vi "GEOM_Bin1DetReadMode.vi"(9 "detectors":T1[](array[typedef]), 10 "Amplifiers":T2[](array[typedef]) {"fliped" items=["none", "horizontal", "vertical"]; "type" items=["LL", "LR", "UL", "UR"]}) -> (1 "detectors out":T1[](array[typedef]))   [LabVIEW 2016]
uses:
  GEOM_Amplifier.ctl
  GEOM_AmpType.ctl
  GEOM_ROI.ctl
  GEOM_Coords.ctl
  GEOM_DetSummaryStruct.ctl
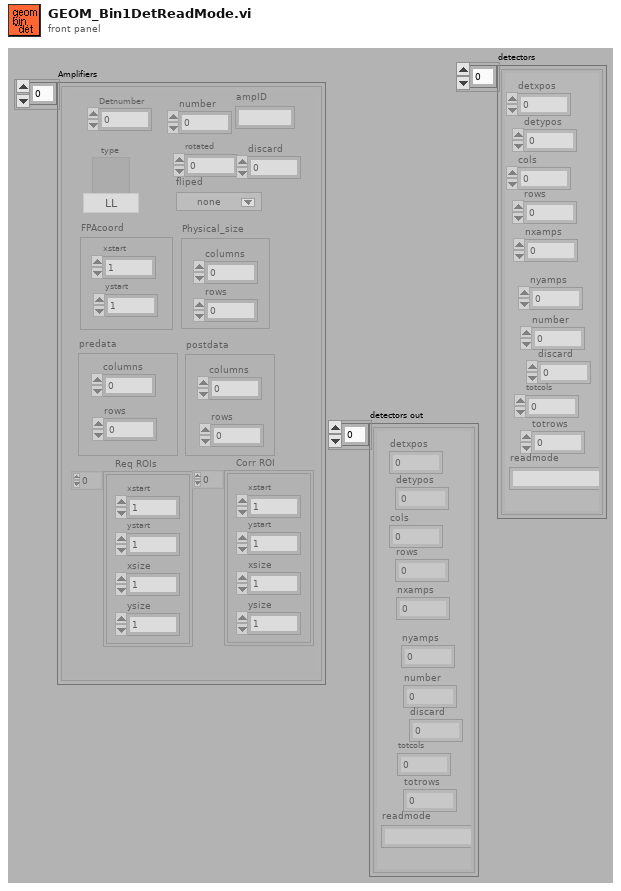
[diagram p1: front panel]
types:
  T1 = typedef "GEOM_DetSummaryStruct.ctl" = cluster{"detxpos":i32, "detypos":i32, "cols":i32, "rows":i32, "nxamps":i32, "nyamps":i32, "number":i32, "discard":i32, "totcols":i32, "totrows":i32, "readmode":string}
  T2 = typedef "GEOM_Amplifier.ctl" = cluster{"number":i32, "type":T3, "rotated":i16, "fliped":u16, "FPAcoord":cluster{"xstart":i32, "ystart":i32}, "Physical_size":cluster{"columns":i32, "rows":i32}, "predata":cluster{"columns":i32, "rows":i32}, "postdata":cluster{"columns":i32, "rows":i32}, "Req ROIs":T4, "Corr ROI":T4, "Detnumber":i32, "ampID":string, "discard":i32}
  T3 = typedef "GEOM_AmpType.ctl" = u16
  T4 = typedef "GEOM_ROI.ctl" = T5[]
  T5 = typedef "GEOM_Coords.ctl" = cluster{"xstart":u32, "ystart":u32, "xsize":u32, "ysize":u32}
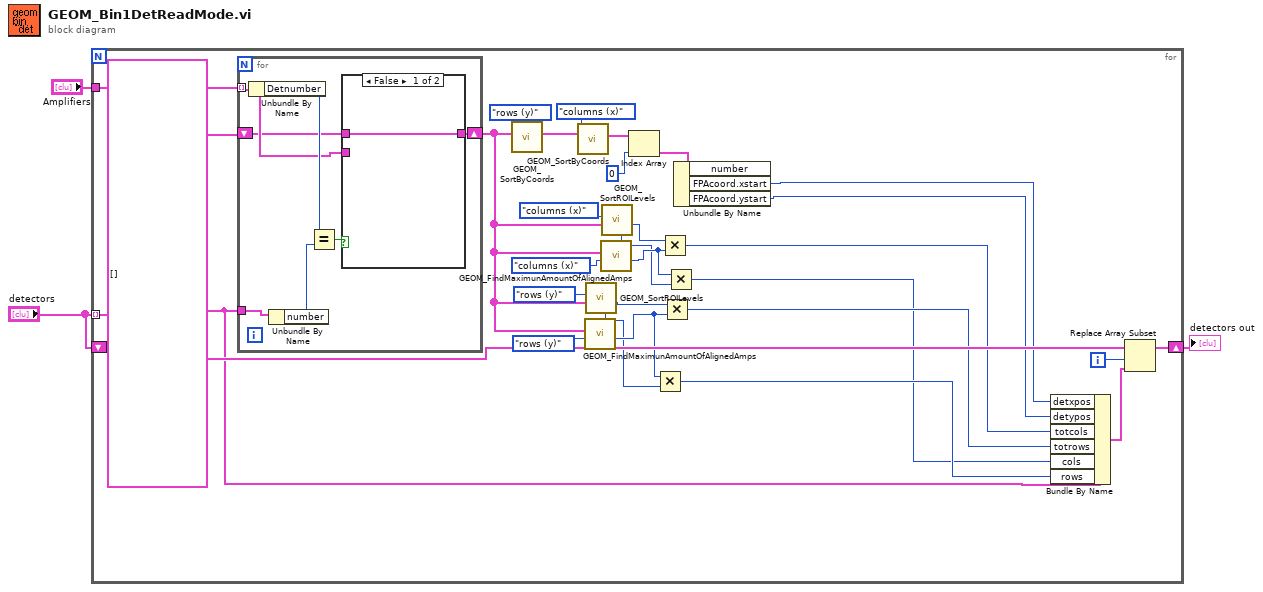
[diagram p0: block diagram]
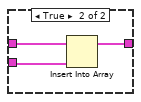
[diagram p2: hidden frame]
diagram:
  n1 = for {
    tunnel: "detectors" -> [w26] mode=indexing
    tunnel: "Amplifiers" -> [w33]
    shift-right: [w24] -> w1
    shift-left: "detectors" -> [w27]
    i -> [w17]
    n2 = for {
      tunnel: w33 -> [w36] mode=indexing
      tunnel: w26 -> [w39]
      shift-right: [w34] -> w18
      shift-left: T2[] [] -> [w35]
      n3 = Unbundle By Name(w36) -> ("Detnumber"=w40:i32)
      n4 = Unbundle By Name(w39) -> ("number"=w38:i32)
      n5 = Equal?(x=w40, y=w38) -> (x = y?=w37:bool)
      n6 = case shown="False" w37 {
        tunnel: w36 -> [_ w43]
        tunnel: [w41 w42] -> w34
        tunnel: w35 -> [w41 w44]
        frame False {
        }
        frame True {
          n7 = Insert Into Array(array=w44, new element=w43) -> (w42:T2[])  [unwired: 1 in]
        }
      }
    }
    n8 = call "GEOM_SortByCoords.vi"("amplifiers"=w18, "how"=enum16{"rows (y)", "columns (x)"}."rows (y)") -> ("sorted amplifiers"=w30:T2[])  [unwired: 9 out]
    n9 = call "GEOM_SortByCoords.vi"("amplifiers"=w30, "how"=enum16{"rows (y)", "columns (x)"}."columns (x)") -> ("sorted amplifiers"=w23:T2[])  [unwired: 9 out]
    n10 = call "GEOM_FindMaximunAmountOfAlignedAmps.vi"("how"=enum16{"rows (y)", "columns (x)"}."rows (y)", "amplifiers"=w18) -> ("maxalignedamps"=w7:i32)  [unwired: 9 out]
    n11 = call "GEOM_SortROILevels.vi"("amplifiers"=w18, "how"=enum16{"rows (y)", "columns (x)"}."rows (y)") -> ("totpix"=w11:u32, "totdata"=w6:i32)  [unwired: 2 in, 6 out]
    n12 = call "GEOM_FindMaximunAmountOfAlignedAmps.vi"("how"=enum16{"rows (y)", "columns (x)"}."columns (x)", "amplifiers"=w18) -> ("maxalignedamps"=w9:i32)  [unwired: 9 out]
    n13 = call "GEOM_SortROILevels.vi"("amplifiers"=w18, "how"=enum16{"rows (y)", "columns (x)"}."columns (x)") -> ("totpix"=w13:u32, "totdata"=w8:i32)  [unwired: 2 in, 6 out]
    n14 = Index Array(array=w23, index=0) -> (element=w16:T2)
    n15 = Multiply(x=w7, y=w6) -> (x*y=w5:i32)
    n16 = Multiply(x=w13, y=w9) -> (x*y=w12:u32)
    n17 = Multiply(x=w11, y=w7) -> (x*y=w10:u32)
    n18 = Multiply(x=w9, y=w8) -> (x*y=w4:i32)
    n19 = Unbundle By Name(w16) -> ("FPAcoord.xstart"=w15:i32, "FPAcoord.ystart"=w14:i32)  [unwired: 1 out]
    n20 = Bundle By Name(cluster=w26, "detxpos"=w15, "detypos"=w14, "totcols"=w12, "totrows"=w10, "cols"=w4, "rows"=w5) -> (w25:T1)
    n21 = Replace Array Subset(array=w27, new element=w25, index=w17) -> (w24:T1[])
  }
  "detectors out" <- w1
